vi "test_cavity_model_constants.vi"   [LabVIEW 2013]
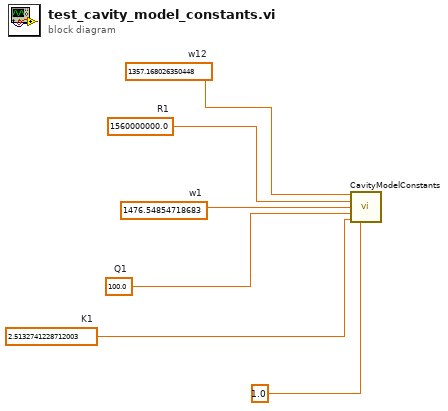
[diagram p0: block diagram]
diagram:
  w2 = 2.5132741228712003  # K1
  w3 = 100.0  # Q1
  w4 = 1476.54854718683  # w1
  w5 = 1560000000.0  # R1
  w6 = 1357.168026350448  # w12
  n1 = call "CavityModelConstants.vi"("w12"=w6, "R1"=w5, "w1"=w4, "Q1"=w3, "K1"=w2, "S"=1.0) -> ()  [unwired: 5 in, 5 out]
